vi "MM9.ReadUserData.vi"(0 "i ref in":refnum<vi>, 1 "Data":string, 3 "timeout ms":i32=10000, 5 "error in (no error)":errorcluster) -> (14 "i ref out":refnum<vi>, 17 "timed out":bool, 19 "error out":errorcluster)   [LabVIEW 2014, in "MM9.lvlib"]
doc: "This method converts raw user data to required configuration information and writes this to the attributes."
uses:
  MM9.lvlib
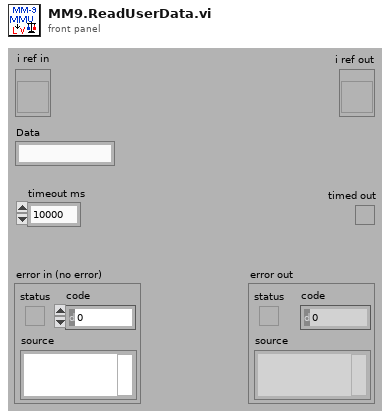
[diagram p1: front panel]
types:
  T1 = typedef "MM9.lvlib/MM9.i attribute.ctl" = cluster{"UsedObjs":string[], "ActScanStep":i32[], "AbortRequest":bool, "StopRequest":bool, "# cycles":i32, "Connected":bool, "MMStatus":T2, "# data":i32, "DIMServices":cluster{"MM6StatusString":string, "MM6StatusID":i32, "discArchiver":string, "discArchiverID":i32, "eventBuilder":string, "eventBuilderID":i32, "GUIIDString":string, "GUIIDStringID":i32}, "dataFile":string, "PGRunning":T3, "ConfigData":T4, "ExtraDataSets":T19}
  T2 = typedef "MM9.lvlib/MM9.status.ctl" = enum16{"loaded", "load_error", "config", "config_error", "init", "init_error", "data_reset", "data_reset_error", "running", "start_error", "run_error", "abort_requested", "aborted", "stop_requested", "stopped", "stop_error", "Connected", "NOTConnected"}
  T3 = typedef "PPG_ABC.lvlib/PPG_ABC.PG_Running.ctl" = i32
  T4 = typedef "LEBITDefs9.lvlib/LEBITDefs.ConfigData.ctl" = cluster{"GenConfig":T5, "Configs":T7[]}
  T5 = typedef "LEBITDefs9.lvlib/LEBITDefs.GenConfig.ctl" = cluster{"Mode":i32, "Logs":T6[]}
  T6 = typedef "LEBITDefs9.lvlib/LEBITDefs.Log.ctl" = cluster{"Name":string, "FctName":string, "Special":string}
  T7 = typedef "LEBITDefs9.lvlib/LEBITDefs.OneConfig.ctl" = cluster{"MCA":T8, "Timing":T9, "Scans":T12[], "FreqDevs":T13[], "CleanDev":T14, "NrCycles":i32, "Specials":T16[], "Delays":T17[], "DAC":T18}
  T8 = typedef "LEBITDefs9.lvlib/LEBITDefs.MCA.ctl" = cluster{"Name":string, "Address":string, "NrChannels":i32, "Gate":i32, "NrPipse":i32, "AcqDelay":i32}
  T9 = typedef "LEBITDefs9.lvlib/LEBITDefs.Timing.ctl" = cluster{"TimeTables":cluster{"TimeTable":T10}[], "Memories":T11[], "ScanX":string, "ScanY":string}
  T10 = typedef "LEBITDefs9.lvlib/LEBITDefs.Timetable.ctl" = dbl[]
  T11 = typedef "LEBITDefs9.lvlib/LEBITDefs.Memory.ctl" = cluster{"Device":string, "ExtTrig":bool, "TT2Use":i32, "PatternTable":string[]}
  T12 = typedef "LEBITDefs9.lvlib/LEBITDefs.ScanDev.ctl" = cluster{"Name":string, "FctName":string, "Values":dbl[], "NrScanVals":i32, "Special":string}
  T13 = typedef "LEBITDefs9.lvlib/LEBITDefs.FreqDev.ctl" = cluster{"Name":string, "Amp":dbl, "CenterFreq":dbl, "Time":dbl}
  T14 = typedef "LEBITDefs9.lvlib/LEBITDefs.CleanDev.ctl" = cluster{"Name":string, "CleanData":T15[]}
  T15 = typedef "LEBITDefs9.lvlib/LEBITDefs.CleanDataType.ctl" = cluster{"Amp":dbl, "Center":dbl, "Plus":dbl, "Minus":dbl, "Time":dbl}
  T16 = typedef "LEBITDefs9.lvlib/LEBITDefs.Special.ctl" = cluster{"Name":string, "FctName":string, "VerySpecial":string, "Data":dbl}
  T17 = typedef "LEBITDefs9.lvlib/LEBITDefs.Delay.ctl" = cluster{"Name":string, "Delay":dbl}
  T18 = typedef "LEBITDefs9.lvlib/LEBITDefs.DAC.ctl" = cluster{"Name":string, "Step1":i32, "Step2":i32}
  T19 = typedef "LEBITDefs9.lvlib/LEBITDefs.ExtraData.ctl" = cluster{"Ions":cluster{"ExcitIonMass":string, "ExcitIonCharge":i32, "CleanIons":cluster{"CleanIonMass":string, "CleanIonCharge":i32}[]}, "TimingDescription":cluster{"TimeTableDescription":cluster{"Times":string[]}[], "PatternTableDescription":cluster{"Pattern":string[]}[]}, "ScanUnits":string[]}[]
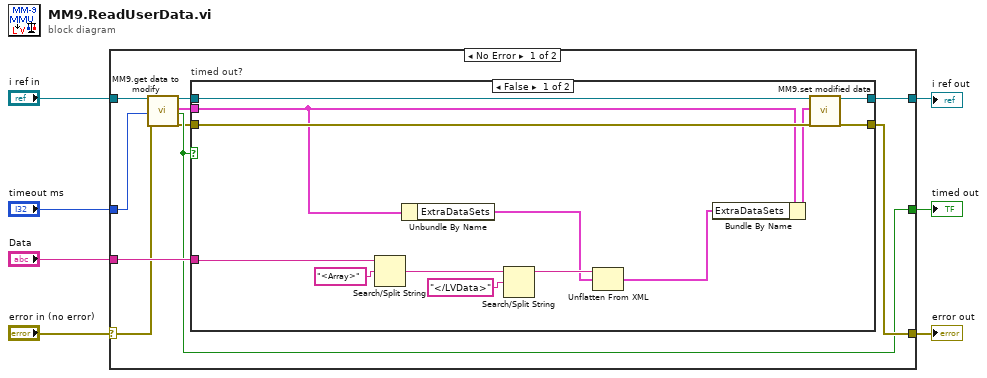
[diagram p0: block diagram]
diagram:
  n1 = case shown="No Error" "error in (no error)" {
    selector: "error in (no error)" -> [w13 w34]
    tunnel: [w17 w34] -> w7
    tunnel: "Data" -> [w16 _]
    tunnel: "i ref in" -> [w15 w33]
    tunnel: "timeout ms" -> [w14 _]
    tunnel: [w12 _] -> w2
    tunnel: [w9 w33] -> w1
    frame No Error {
      n2 = call "MM9.get data to modify.vi"("i ref in"=w15, "ms timeout (10000)"=w14, "error in (no error)"=w13) -> ("i ref out"=w10:refnum<vi>, "i attribute"=w8:T1, "timed out"=w12:bool, "error out"=w11:errorcluster)  [unwired: 13 in]
      n3 = case "timed out?" shown="False" w12 {
        tunnel: [w28 w32] -> w17
        tunnel: w16 -> [w26 _]
        tunnel: w11 -> [w27 w32]
        tunnel: w10 -> [w30 w31]
        tunnel: [w29 w31] -> w9
        tunnel: w8 -> [w25 _]
        frame False {
          n4 = Search/Split String(string=w26, search string/char (-)="<Array>") -> (match + rest of string=w22:string)  [unwired: 1 in, 2 out]
          n5 = Unbundle By Name(w25) -> ("ExtraDataSets"=w18:T19)
          n6 = Search/Split String(string=w22, search string/char (-)="</LVData>") -> (substring before match=w19:string)  [unwired: 1 in, 2 out]
          n7 = Unflatten From XML(xml string=w19, type=w18) -> (value=w23:T19)  [unwired: 1 in, 1 out]
          n8 = Bundle By Name(cluster=w25, "ExtraDataSets"=w23) -> (w24:T1)
          n9 = call "MM9.set modified data.vi"("i ref in"=w30, "i attribute"=w24, "error in (no error)"=w27) -> ("i ref out"=w29:refnum<vi>, "error out"=w28:errorcluster)  [unwired: 15 in]
        }
        frame True {
        }
      }
    }
    frame Error {
    }
  }
  "error out" <- w7
  "i ref out" <- w1
  "timed out" <- w2
